vi "读取配置文件引用 i.vi"(8 "error in (no error)":errorcluster caption="错误输入（无错误）", 11 "配置文件-输入":refnum<class "配置文件-.lvclass">) -> (0 "error out":errorcluster caption="错误输出", 2 "config data":T1 caption="配置数据", 3 "配置文件-输出":refnum<class "配置文件-.lvclass">)   [LabVIEW 2017, in "项目开发助手.lvlib" / "模板-配置文件相关.lvlib" / "配置文件-.lvclass"]
uses:
  <vilib>/Utility/config.llb/Config Data RefNum.ctl
  <vilib>/Utility/config.llb/NI_LVConfig.lvlib
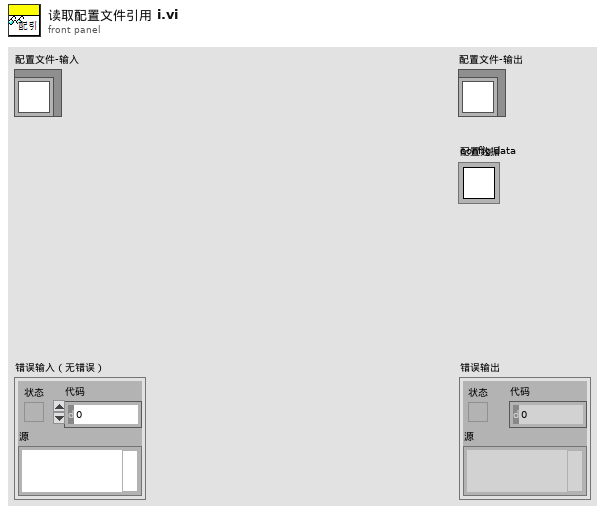
[diagram p1: front panel]
types:
  T1 = typedef "NI_LVConfig.lvlib/Config Data RefNum.ctl" = refnum<k1>
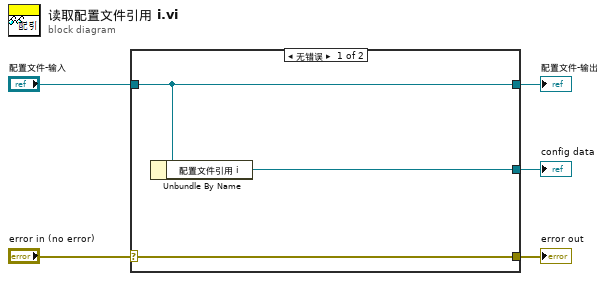
[diagram p0: block diagram]
diagram:
  n1 = case shown="无错误" "error in (no error)" {
    selector: "error in (no error)" -> [w8 w9]
    tunnel: [w8 w9] -> w4
    tunnel: [w7 w10] -> w2
    tunnel: "配置文件-输入" -> [w7 w10]
    tunnel: [w6 _] -> w1
    frame No Error {
      n2 = Unbundle By Name(w7) -> ("配置文件引用 i"=w6:T1)
    }
    frame Error {
    }
  }
  "error out" <- w4
  "配置文件-输出" <- w2
  "config data" <- w1
